vi "MV3D RGBD Open Device By Ip.vi"(10 "chIP":string, 11 "handle":u32) -> (2 "function return":i32, 3 "handle out":u32)   [LabVIEW 2015, in "Mv3dRgbd.lvlib"]
doc: "MV3D_RGBD_API MV3D_RGBD_STATUS MV3D_RGBD_OpenDeviceByIp(HANDLE *handle, const char* chIP);"
uses:
  <userlib>/Mv3dRgbd/Mv3dRgbd.lvlib
  <userlib>/Mv3dRgbd/Mv3dRgbd.dll
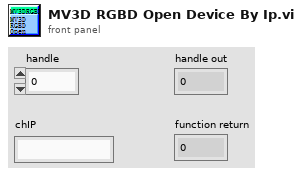
[diagram p1: front panel]
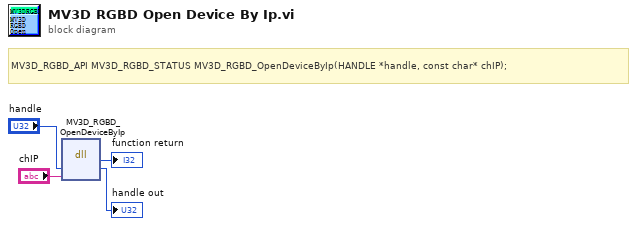
[diagram p0: block diagram]
diagram:
  # "MV3D_RGBD_API MV3D_RGBD_STATUS MV3D_RGBD_OpenDeviceByIp(HANDLE *handle, const char* chIP);"
  n1 = dll-call lib="C:/Program Files (x86)/National Instruments/LabVIEW 2015/user.lib/Mv3dRgbd/Mv3dRgbd.*" fn="MV3D_RGBD_OpenDeviceByIp"("handle"="handle", "chIP"="chIP") -> (→"function return":i32, "handle"=→"handle out":u32)  [unwired: 4 in, 2 out]
